vi "Measure Events.vi"   [LabVIEW 2013, in "Engine Simulation Toolkit.lvlib" / "ECU Event Timing.lvlib"]
doc: "Measures the characteristics of digital events (pulses) within a given angular position window. Combine this VI with 1 or more Event Capture.vi's to send event measurement data up to NI VeriStand. \n\nTo save FPGA resources, select the 40 MHz version of this VI when you place this VI inside a single cycle timed loop operating at 40 MHz. If this VI is inside a while loop, or a single cycle timed loop inside a while loop, select the Non-40 MHz version of this VI.\n\n<b>settings.<user name></b> - settings for the component. NI VeriStand will set these values. Create a control for this input. Replace <user name> with the name you wish this component to display as inside NI VeriStand. Make this name consistent for all controls, indicators, for all VIs of this component.\n<b>event</b> - digital event (pulse) to measure. Can be active high or active low, NI VeriStand has a setting for configuring this.\n<b>register bus</b> - connect this input to the output of the initialize APU VI. This contains references to APU state variables like position and speed.\n\n<b>status.<user name></b> - output for the component. NI VeriStand will read these values. Create an indicator for this output. Replace <user name> with the name you wish this component to display as inside NI VeriStand. Make this name consistent for all controls, indicators, for all VIs of this component.\n<b>measured data</b> - event data to be wired to the Capture Event.vi"
uses:
  ECU Event Timing.lvlib
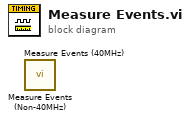
[diagram p0: block diagram]
diagram:
  n1 = call "Measure Events (Non-40MHz).vi"() -> ()  [unwired: 10 in, 2 out]
  n2 = call "Measure Events (40MHz).vi"() -> ()  [unwired: 10 in, 2 out]
